vi "DWF MSO Configure Analog Channel.vi"(0 "Instrument Handle In":u32, 1 "Enable Channel":bool=TRUE caption="Enable Channel (no change)", 5 "Channel":string, 7 "Vertical Coupling":i32(ring)=1 items=["AC", "DC"], 9 "Probe Attenuation":i32(ring)=1 items=["1x"=1, "10x"=10], 11 "Error In":errorcluster caption="Error In (no error)", 12 "Vertical Range":dbl=1.0, 13 "Vertical Offset":dbl) -> (4 "Instrument Handle Out":u32, 15 "Error Out":errorcluster)   [LabVIEW 2015, in "DigilentWF.lvlib"]
doc: "Configures the settings of the specified analog channel."
uses:
  <vilib>/DigilentWF/DigilentWF.lvlib
  dwf.dll
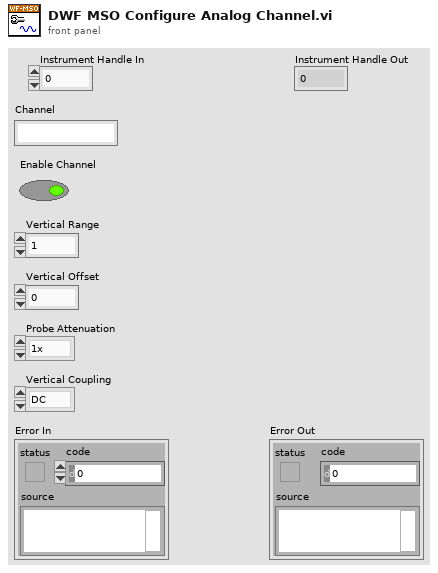
[diagram p1: front panel]
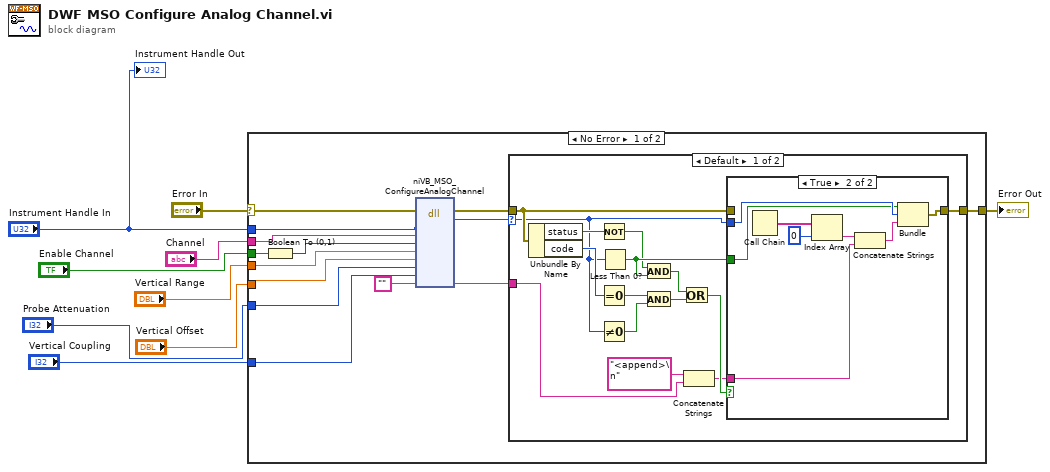
[diagram p0: block diagram]
diagram:
  n1 = case "outter_case" shown="No Error" "Error In" {
    selector: "Error In" -> [w21 w49]
    tunnel: [w23 w49] -> w8
    tunnel: "Instrument Handle In" -> [w19 _]
    tunnel: "Channel" -> [w18 _]
    tunnel: "Enable Channel" -> [w22 _]
    tunnel: "Vertical Range" -> [w16 _]
    tunnel: "Vertical Offset" -> [w15 _]
    tunnel: "Probe Attenuation" -> [w14 _]
    tunnel: "Vertical Coupling" -> [w13 _]
    frame No Error {
      n2 = Boolean To (0,1)(Boolean=w22) -> (0, 1=w17:i16)
      n3 = dll-call lib="dwf.*" fn="niVB_MSO_ConfigureAnalogChannel"(error in=w21, "instrumentHandle"=w19, "channel"=w18, "enableChannel"=w17, "verticalRange"=w16, "verticalOffset"=w15, "probeAttenuation"=w14, "verticalCoupling"=w13, "szError"="") -> (error out=w20:errorcluster, "return type"=w12:i32, "szError"=w10:string)  [unwired: 9 in, 1 out]
      n4 = case "inner_case" shown="Default" w12 {
        selector: w12 -> [w28 _]
        tunnel: w20 -> [w29 w48]
        tunnel: [w25 w48] -> w23
        tunnel: w10 -> [w24 _]
        frame Default {
          n5 = Unbundle By Name(w29) -> ("status"=w33:bool, "code"=w37:i32)
          n6 = Not(x=w33) -> (.not. x?=w36:bool)
          n7 = Equal To 0?(x=w37) -> (x = 0?=w32:bool)
          n8 = Not Equal To 0?(x=w28) -> (x != 0?=w35:bool)
          n9 = Less Than 0?(x=w28) -> (x < 0?=w38:bool)
          n10 = And(x=w36, y=w38) -> (x .and. y?=w34:bool)
          n11 = And(x=w32, y=w35) -> (x .and. y?=w31:bool)
          n12 = Or(x=w34, y=w31) -> (x .or. y?=w30:bool)
          n13 = Concatenate Strings("<append>\n" ("string"), w24) -> (w27:string)
          n14 = case shown="True" w30 {
            tunnel: [w39 w46] -> w25
            tunnel: w28 -> [_ w45]
            tunnel: w38 -> [_ w44]
            tunnel: w29 -> [w39 _]
            tunnel: w27 -> [_ w40]
            frame False {
            }
            frame True {
              n15 = Call Chain() -> (call chain=w43:string[])
              n16 = Index Array(array=w43, index=0) -> (element=w42:string)
              n17 = Concatenate Strings(w42, w40) -> (w47:string)
              n18 = Bundle(w44, "return type"=w45, w47) -> (w46:cluster{bool, "return type":i32, string})  [unwired: 1 out]
            }
          }
        }
        frame 0 {
        }
      }
    }
    frame Error {
    }
  }
  "Error Out" <- w8
  "Instrument Handle Out" <- "Instrument Handle In"
